vi "Configure Marker Trace (Burst Power).vi"(6 "Enable Min Hold Trace (F: Disable)":bool, 7 "Enable Max Hold Trace (F: Disable)":bool, 8 "error in (no error)":errorcluster, 9 "Marker Trace (0: RF Envelope)":i32(ring) items=["RF Envelope", "Max Hold RF Envelope", "Min Hold RF Envelope"], 10 "Active Marker (1: Marker1)":i32(ring)=1 items=["Marker1"=1, "Marker2"=2, "Marker3"=3, "Marker4"=4, "Marker5"=5, "Marker6"=6, "Marker7"=7, "Marker8"=8, "Marker9"=9, "Marker10"=10, "Marker11"=11, "Marker12"=12], 11 "VISA resource name":refnum<visa-resource-name>) -> (0 "error out":errorcluster, 3 "VISA resource name out":refnum<visa-resource-name>)   [LabVIEW 2014, in "Agilent MXA Series.lvlib"]
doc: "Selects the trace that you want your marker to be placed on under Burst Power measurement type."
uses:
  Agilent MXA Series.lvlib
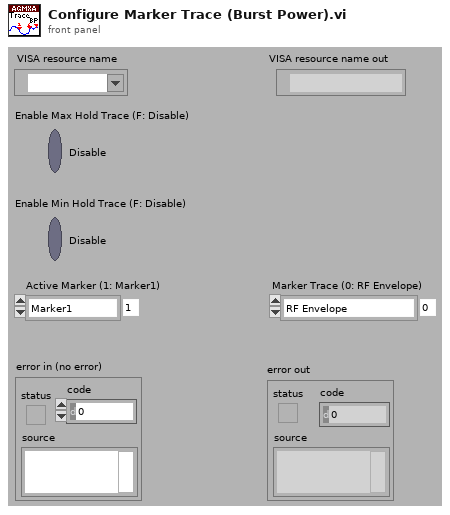
[diagram p1: front panel]
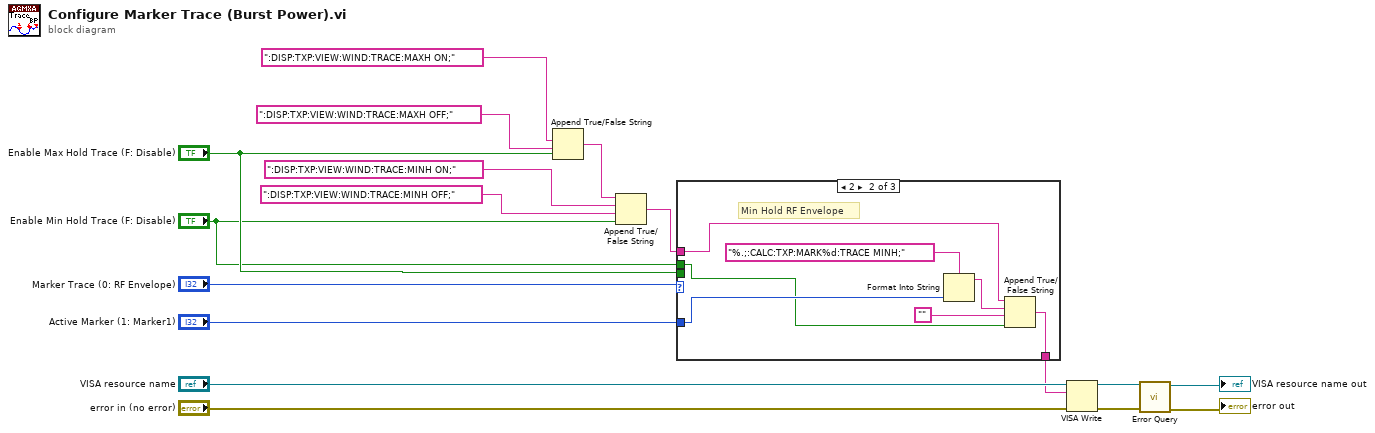
[diagram p0: block diagram]
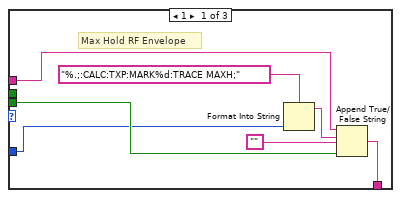
[diagram p2: hidden frame]
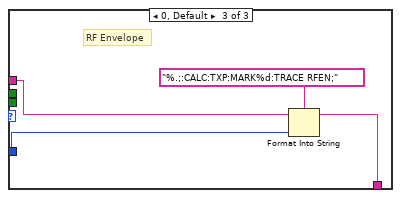
[diagram p3: hidden frame]
diagram:
  n1 = Append True/False String(1:"Enable Max Hold Trace (F: Disable)", 2:":DISP:TXP:VIEW:WIND:TRACE:MAXH OFF;" ("false string"), 3:":DISP:TXP:VIEW:WIND:TRACE:MAXH ON;" ("true string")) -> (0:w13:string)  [unwired: 1 in]
  n2 = Append True/False String(1:"Enable Min Hold Trace (F: Disable)", 2:":DISP:TXP:VIEW:WIND:TRACE:MINH OFF;" ("false string"), 3:":DISP:TXP:VIEW:WIND:TRACE:MINH ON;" ("true string"), 4:w13) -> (0:w8:string)
  n3 = case shown="2" "Marker Trace (0: RF Envelope)" {
    tunnel: "Active Marker (1: Marker1)" -> [w23 w31 w35]
    tunnel: w8 -> [w18 w25 w33]
    tunnel: [w19 w27 w32] -> w5
    tunnel: "Enable Max Hold Trace (F: Disable)" -> [w24 _ _]
    tunnel: "Enable Min Hold Trace (F: Disable)" -> [_ w26 _]
    frame 1 {
      # "Max Hold RF Envelope"
      n4 = Format Into String(format string="%.;:CALC:TXP:MARK%d:TRACE MAXH;", w23) -> (resulting string=w21:string)  [unwired: 2 in, 1 out]
      n5 = Append True/False String(1:w24, 2:"", 3:w21, 4:w18) -> (0:w19:string)
    }
    frame 2 {
      # "Min Hold RF Envelope"
      n6 = Format Into String(format string="%.;:CALC:TXP:MARK%d:TRACE MINH;", w31) -> (resulting string=w29:string)  [unwired: 2 in, 1 out]
      n7 = Append True/False String(1:w26, 2:"", 3:w29, 4:w25) -> (0:w27:string)
    }
    frame 0, Default {
      # "RF Envelope"
      n8 = Format Into String(format string="%.;:CALC:TXP:MARK%d:TRACE RFEN;", initial string=w33, w35) -> (resulting string=w32:string)  [unwired: 1 in, 1 out]
    }
  }
  n9 = VISA Write(VISA resource name="VISA resource name", write buffer=w5, error in (no error)="error in (no error)") -> (VISA resource name out=w4:refnum<visa-resource-name>, error out=w2:errorcluster)  [unwired: 1 out]
  n10 = call "Error Query.vi"("error in (no error)"=w2, "VISA resource name"=w4) -> ("error out"=→"error out":errorcluster, "VISA resource name out"=→"VISA resource name out":refnum<visa-resource-name>)  [unwired: 6 in, 2 out]
